vi "ip address.vi"() -> (3 "ip address":string)   [LabVIEW 2014]
uses:
  <vilib>/regexp/Match Regular Expression.xnode
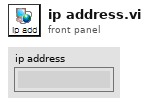
[diagram p1: front panel]
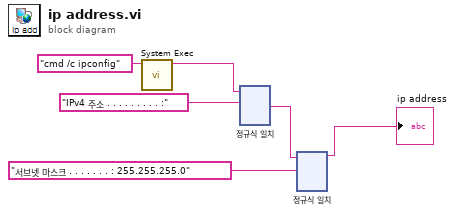
[diagram p0: block diagram]
diagram:
  n1 = call <vilib>:"System Exec.vi"("command line"="cmd /c ipconfig") -> ("standard output"=w5:string)  [unwired: 7 in, 3 out]
  n2 = xnode "정규식 일치"("입력 문자열"=w5, "정규식"="IPv4 주소 . . . . . . . . . :") -> ("일치 구문 뒤"=w3:string)  [unwired: 4 in, 4 out]
  n3 = xnode "정규식 일치"("입력 문자열"=w3, "정규식"="서브넷 마스크 . . . . . . . : 255.255.255.0") -> ("일치 구문 앞"=→"ip address":string)  [unwired: 4 in, 4 out]
